vi "Launcher.vi"   [LabVIEW 2020]
uses:
  User Interface/User Interface.lvclass
  <vilib>/ActorFramework/Actor/Actor.lvclass
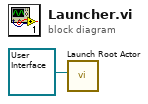
[diagram p0: block diagram]
diagram:
  n1 = call <vilib>:"Launch Root Actor.vi"("Actor"=refnum<class "User Interface.lvclass"> refnum ("User Interface.lvlib:User Interface.lvclass")) -> ()  [unwired: 9 in, 2 out]
